vi "VI Server_Get Control Label_Refernce_Value_StringFormat.vi"(7 "Label":string, 8 "error in (no error)":errorcluster, 11 "VI Server Cluster":T1) -> (0 "error out":errorcluster, 1 "ControlValue(StringFormat)":string, 3 "VI Server Cluster.DUP":T1)   [LabVIEW 2020]
doc: "Returns control's value formatted as string.\nUsed for saving such values into configuration file."
uses:
  VI Server_TypeDefs/VI Server_RefsCluster.ctl
  VI Server Libraries/VI Server Controls.llb/VI Server_GetSet Controls From String Format_Options.ctl
  VI Server Toolkit LV2013.lvlib
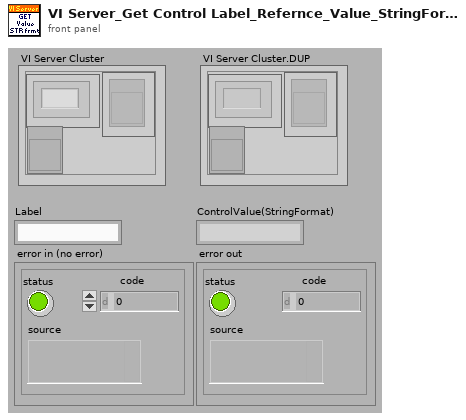
[diagram p1: front panel]
types:
  T1 = typedef "VI Server_RefsCluster.ctl" = cluster{"Labels":string[], "Refs":refnum<vi>[], "VI Ref":refnum<vi>}
  T2 = typedef "VI Server Toolkit LV2013.lvlib/VI Server_GetSet Controls From String Format_Options.ctl" = enum16{"", "If Ring Get Selection", "If Ring Set by Selection"}
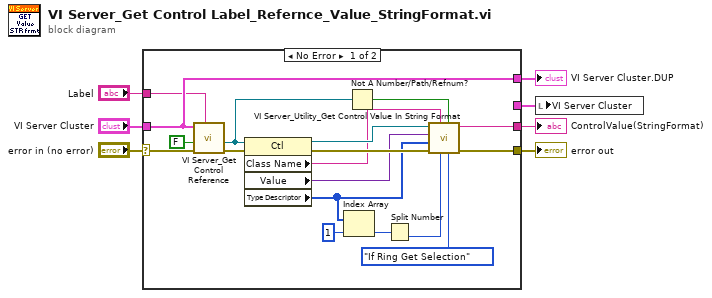
[diagram p0: block diagram]
diagram:
  n1 = case shown="No Error" "error in (no error)" {
    selector: "error in (no error)" -> [w23 w27]
    tunnel: [w16 w27] -> w7
    tunnel: "VI Server Cluster" -> [w21 _]
    tunnel: "Label" -> [w20 _]
    tunnel: [w9 _] -> w3
    tunnel: [w21 _] -> w2
    tunnel: [_ w26] -> w1
    frame No Error {
      n2 = call "VI Server_Get Control Reference.vi"("Label"=w20, "error in"=w23, "Single Instance (T)"=FALSE, "VI Server Cluster"=w21) -> ("error out"=w22:errorcluster, "Control Reference (Generic)"=w19:refnum<vi>)  [unwired: 4 in, 2 out]
      n3 = property class="Ctl"(reference=w19, error in=w22) -> (reference out=w15:refnum<vi>, error out=w17:errorcluster, "Class Name"=w13:string, "Value"=w12:variant, "Type Descriptor"=w10:i16[])
      n4 = Index Array(array=w10, index=1) -> (element=w24:i16)
      n5 = Not A Number/Path/Refnum?(number/path/refnum=w19) -> (NaN/Path/Refnum?=w14:bool)
      n6 = Split Number(x=w24) -> (lo(x)=w11:u8)  [unwired: 1 out]
      n7 = call "VI Server_Utility_Get Control Value In String Format.vi"("Options"=VI_Server_GetSet_Controls_From_String_Format_Options."If Ring Get Selection", "Continue"=w14, "Control.Representation"=w11, "Control.ClassName"=w13, "error in (no error)"=w17, "TypeDesc"=w10, "Control.Value.Invariant"=w12, "Control.Ref"=w15) -> ("error out"=w16:errorcluster, "Control.String.OUT"=w9:string)  [unwired: 2 out]
    }
    frame Error {
      n8 = call "VI Server_Empty VI Server Cluster.vi"() -> ("VI Server Cluster"=w26:T1)  [unwired: 7 in]
    }
  }
  "error out" <- w7
  "VI Server Cluster.DUP" <- w2
  "ControlValue(StringFormat)" <- w3
  n9 = local write "VI Server Cluster"(w1) -> ()
